vi "Camera Init mk1.vi"(2 "Image Name":string="Image") -> (0 "error out":errorcluster, 1 "IMAQ USB Session Out":T1, 3 "New Image":T2)   [LabVIEW 2011]
uses:
  <vilib>/vision/Image Controls.llb/IMAQ Image.ctl
  <vilib>/imaqUSB/imaqUSB.llb/IMAQ USB.ctl
  <vilib>/vision/NI_Vision_Development_Module.lvlib
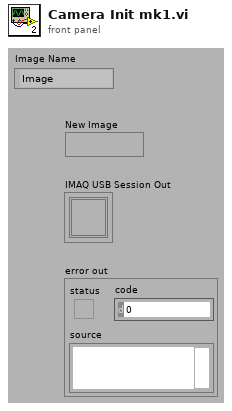
[diagram p1: front panel]
types:
  T1 = typedef "IMAQ USB.ctl" = refnum<k1>
  T2 = typedef "IMAQ Image.ctl" = refnum<image>
  T3 = typedef "Image Type" = u32
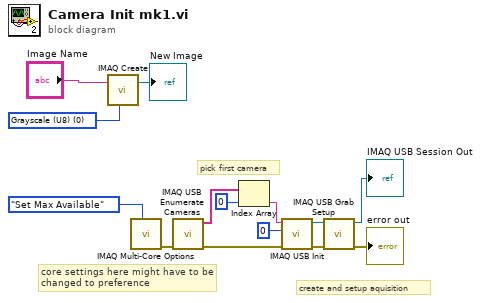
[diagram p0: block diagram]
diagram:
  w13 = T3 0 items=["Grayscale (U8)", "Grayscale (I16)", "Grayscale (SGL)", "Complex (CSG)", "RGB (U32)", "HSL (U32)", "RGB (U64)", "Grayscale (U16)"] ("Image Type")
  # "create and setup aquisition"
  # "core settings here might have to be \nchanged to preference"
  # "pick first camera"
  n1 = call "IMAQ Create"("Image Name"="Image Name", "Image Type"=w13) -> ("New Image"=→"New Image":T2)  [unwired: 2 in, 2 out]
  n2 = call "IMAQ Multi-Core Options"("Get/Set Number of Cores (Get)"=enum32{"Get", "Set", "Set Max Available"}."Set Max Available") -> ("error out"=w10:errorcluster)  [unwired: 2 in, 8 out]
  n3 = call <vilib>:"IMAQ USB Enumerate Cameras.vi"("error in (no error)"=w10) -> ("error out"=w5:errorcluster, "USB Camera Names"=w3:string[])  [unwired: 9 out]
  n4 = Index Array(array=w3, index=0) -> (element=w4:string)
  n5 = call <vilib>:"IMAQ USB Init.vi"("error in (no error)"=w5, "Video Mode"=0, "USB Camera Name"=w4) -> ("error out"=w6:errorcluster, "IMAQ USB Session Out"=w7:T1)  [unwired: 7 out]
  n6 = call <vilib>:"IMAQ USB Grab Setup.vi"("error in (no error)"=w6, "IMAQ USB Session In"=w7) -> ("error out"=→"error out":errorcluster, "IMAQ USB Session Out"=→"IMAQ USB Session Out":T1)  [unwired: 8 out]
